vi "unbundleByNameProgrammatically.vi"(8 "error in (no error)":errorcluster, 9 "Value":variant, 10 "Name":string, 11 "Cluster Ref In":refnum<vi>) -> (0 "error out":errorcluster, 3 "Cluster Ref Out":refnum<vi>)   [LabVIEW 2012]
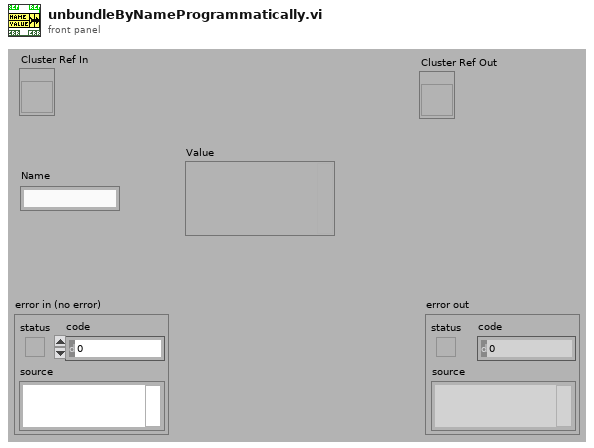
[diagram p1: front panel]
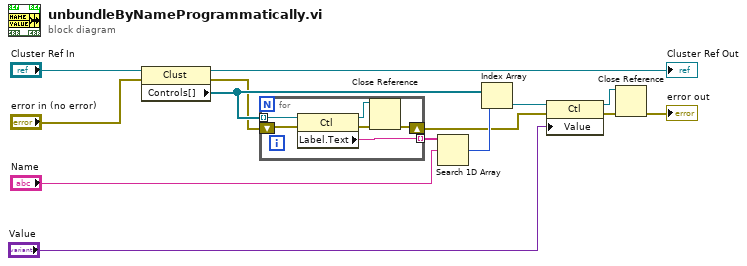
[diagram p0: block diagram]
diagram:
  n1 = property class="Clust"(reference="Cluster Ref In", error in="error in (no error)") -> (reference out=→"Cluster Ref Out":refnum<vi>, error out=w9:errorcluster, "Controls[]"=w12:refnum<vi>[])
  n2 = for {
    tunnel: w12 -> [w20] mode=indexing
    tunnel: [w19] -> w11 mode=indexing
    shift-right: [w15] -> w2
    shift-left: w9 -> [w16]
    n3 = property class="Ctl"(reference=w20, error in=w16) -> (reference out=w17:refnum<vi>, error out=w18:errorcluster, "Label.Text"=w19:string)
    n4 = Close Reference(reference=w17, error in (no error)=w18) -> (error out=w15:errorcluster)
  }
  n5 = Search 1D Array(1D array=w11, element="Name") -> (index of element=w7:i32)  [unwired: 1 in]
  n6 = Index Array(array=w12, index=w7) -> (element=w6:refnum<vi>)
  n7 = property class="Ctl"(reference=w6, error in=w2, "Value"="Value") -> (reference out=w4:refnum<vi>, error out=w5:errorcluster)
  n8 = Close Reference(reference=w4, error in (no error)=w5) -> (error out=→"error out":errorcluster)
